vi "(Var) Get_HVPS_3.vi"() -> ()   [LabVIEW 2017]
panel:
  out "G3. Q Stop":bool=TRUE
  out "G3. Stop":bool=TRUE
  out "G3. Start":bool=TRUE
  out "G3. Error ?":bool
  out "G3. mA":dbl
  out "G3. KV":dbl
  out "G3. Read Mode":string
  out "G3. Read HV":string
  out "G3. Read State":string
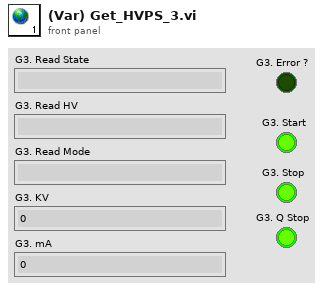
[diagram p1: front panel]
diagram:
